vi "Rename Classes.vi"(8 "error in (no error)":errorcluster, 11 "ProjectItem in":refnum<class "ProjectItem.lvclass">) -> (0 "error out":errorcluster, 3 "ProjectItem out":refnum<class "ProjectItem.lvclass">)   [LabVIEW 2019, in "ProjectItem.lvclass"]
uses:
  ProjectItem.lvclass
  ProjectItem.lvclass/ProjectItem.ctl
panel:
  out "Class Names":string[](array[string])
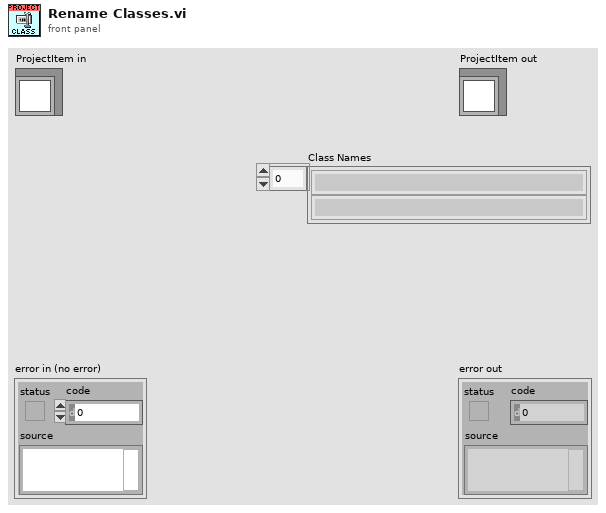
[diagram p1: front panel]
types:
  T1 = cluster{"Class":refnum<vi>, "DynamicVIs":refnum<vi>[], "StaticVIs":refnum<vi>[], "Controls":refnum<vi>[], "Name":string, "Icon":refnum<class "Icon.lvclass">, "Wire Foreground Color":u32}[]
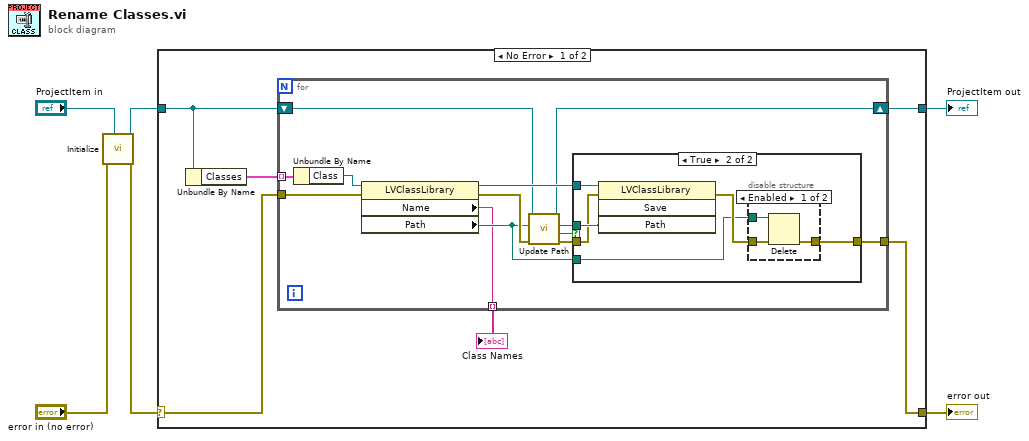
[diagram p0: block diagram]
diagram:
  n1 = call "Initialize.vi"("ProjectItem"="ProjectItem in", "error in (no error)"="error in (no error)") -> ("error out"=w1:errorcluster, "ProjectItem out"=w3:refnum<class "ProjectItem.lvclass">)  [unwired: 8 in]
  n2 = case shown="No Error" w1 {
    selector: w1 -> [w7 w38]
    tunnel: [w12 w38] -> w6
    tunnel: [w10 w37] -> w5
    tunnel: w3 -> [w8 w37]
    frame No Error {
      n3 = Unbundle By Name(w8) -> ("Classes"=w9:T1)
      n4 = for {
        tunnel: [w22] -> w12
        tunnel: [w18] -> w11 mode=indexing
        tunnel: w9 -> [w16] mode=indexing
        tunnel: w7 -> [w17]
        shift-right: [w13] -> w10
        shift-left: w8 -> [w14]
        n5 = Unbundle By Name(w16) -> ("Class"=w15:refnum<vi>)
        n6 = property class="LVClassLibrary"(reference=w15, error in=w17) -> (reference out=w25:refnum<vi>, error out=w20:errorcluster, "Name"=w18:string, "Path"=w19:path)
        n7 = call "Update Path.vi"("error in (no error)"=w20, "Path in"=w19, "Rename in"=w14) -> ("error out"=w24:errorcluster, "New Path?"=w21:bool, "Path out"=w23:path, "Rename out"=w13:refnum<class "ProjectItem.lvclass">)  [unwired: 5 in]
        n8 = case shown="True" w21 {
          tunnel: w25 -> [_ w32]
          tunnel: w24 -> [w26 w27]
          tunnel: w23 -> [_ w31]
          tunnel: [w26 w29] -> w22
          tunnel: w19 -> [_ w28]
          frame False {
          }
          frame True {
            n9 = invoke class="LVClassLibrary" method="Save"(reference=w32, error in=w27, "Path"=w31) -> (error out=w30:errorcluster)  [unwired: 1 in, 3 out]
            n10 = disable-structure shown="Enabled" {
              disable-tunnel: w28 -> [w35 _]
              disable-tunnel: w30 -> [w34 w36]
              disable-tunnel: [w33 w36] -> w29
              frame Enabled {
                n11 = Delete(path (use dialog)=w35, error in=w34) -> (error out=w33:errorcluster)  [unwired: 3 in, 2 out]
              }
              frame Disabled {
              }
            }
          }
        }
      }
      "Class Names" <- w11
    }
    frame Error {
    }
  }
  "error out" <- w6
  "ProjectItem out" <- w5
